vi "Echo.vi"(8 "error in (no error)":errorcluster, 10 "Error In":errorcluster, 11 "Level3Handler in":refnum<class "Level3Handler.lvclass">) -> (0 "error out":errorcluster, 1 "Still Pass?":bool, 2 "handled?":bool, 3 "Level3Handler out":refnum<class "Level3Handler.lvclass">)   [LabVIEW 2014, in "Chain Of Responsibility Pattern.lvlib" / "Level3Handler.lvclass"]
uses:
  Level3Handler.lvclass
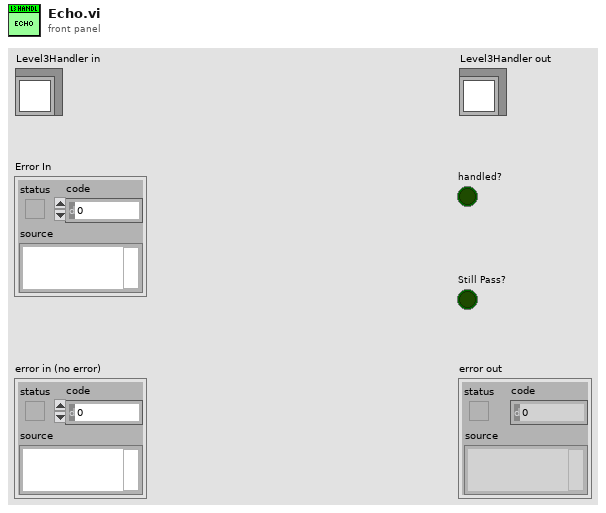
[diagram p1: front panel]
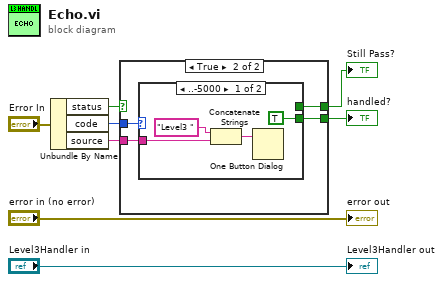
[diagram p0: block diagram]
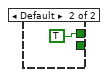
[diagram p3: hidden frame]
diagram:
  n1 = Unbundle By Name("Error In") -> ("status"=w6:bool, "code"=w8:i32, "source"=w7:string)
  n2 = case shown="True" w6 {
    tunnel: w8 -> [_ w12]
    tunnel: [_ w11] -> w1
    tunnel: w7 -> [_ w10]
    tunnel: [_ w9] -> w2
    frame False {
    }
    frame True {
      n3 = case shown="..-5000" w12 {
        tunnel: [_ TRUE] -> w11
        tunnel: w10 -> [w16 _]
        tunnel: [TRUE _] -> w9
        frame ..-5000 {
          n4 = Concatenate Strings("Level3 " ("string"), w16) -> (w15:string)
          n5 = One Button Dialog(message=w15) -> ()  [unwired: 1 in, 1 out]
        }
        frame Default {
        }
      }
    }
  }
  "Still Pass?" <- w1
  "handled?" <- w2
  "error out" <- "error in (no error)"
  "Level3Handler out" <- "Level3Handler in"
